vi "WLAN Tx Test Get Default LSL.vi"(8 "error in (no error)":errorcluster, 11 "Template Tx Test in":refnum<class "niDTS WLAN Tx Test.lvclass">) -> (0 "error out":errorcluster, 2 "Default LSL":T1 {"OBW"."Stop Frequency (Hz)" format="%#_4p"; "OBW"."Start Frequency (Hz)" format="%#_4p"; "OBW"."OBW (Hz)" format="%#_4p"}, 3 "Template Tx Test out":refnum<class "niDTS WLAN Tx Test.lvclass">)   [LabVIEW 2015, in "niDTS WLAN.lvlib" / "niDTS WLAN Tx Test.lvclass"]
uses:
  niDTS WLAN Tx Test.lvclass
  Includes/niDTS WLAN Tx Test INC Results.ctl
  Includes/niDTS WLAN Tx Test INC MOD EVM Results.ctl
  Includes/Results/niDTS Tx RES INC EVM.ctl
  Includes/niDTS WLAN Tx Test INC TXP Results.ctl
  Includes/niDTS WLAN Tx Test INC TXP Result SINGLE.ctl
  Includes/niDTS WLAN Tx Test INC OBW Results.ctl
  Instrument/INSTR TX/Results/niDTS WLAN INSTR TX INC SEM Results.ctl
  Instrument/INSTR TX/Results/niDTS WLAN INSTR TX INC SEM FSEGemts Results.ctl
  Includes/Results/niDTS Tx RES INC SEM FSEGemts.ctl
  Instrument/INSTR TX/Results/niDTS WLAN INSTR TX INC SEM MARGin Results.ctl
  Includes/Results/niDTS Tx RES INC SEM Margin.ctl
  Instrument/INSTR TX/Results/niDTS WLAN INSTR TX INC OFDM Impairments Results.ctl
  niDTS WLAN Tx Test.lvclass/niDTS WLAN Tx Test.ctl
  Includes/niDTS WLAN Tx Test INC Default Limits.vi
  niDTS WLAN.lvlib
  Instrument/INSTR TX/niDTS WLAN INSTR TX.lvclass
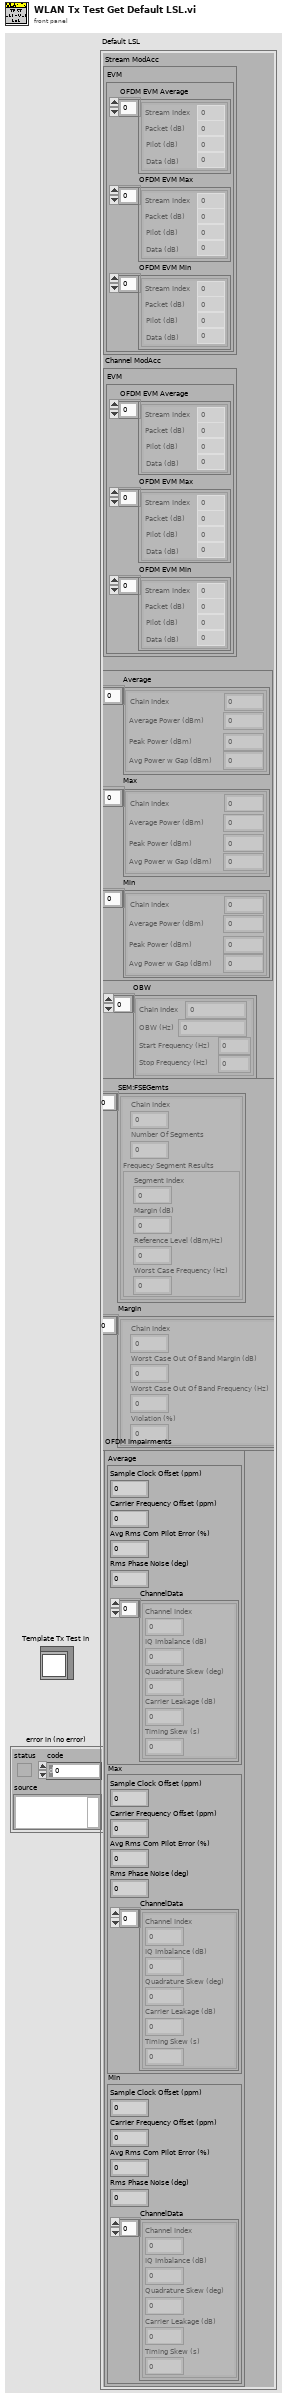
[diagram p1: front panel]
types:
  T1 = typedef "niDTS WLAN.lvlib/niDTS WLAN Tx Test INC Results.ctl" = cluster{"Stream ModAcc":T2, "Channel ModAcc":T2, "TXP":T4, "OBW":T6[], "SEM Results":T7, "OFDM Impairments":T12}
  T2 = typedef "niDTS WLAN.lvlib/niDTS WLAN Tx Test INC MOD EVM Results.ctl" = cluster{"EVM":cluster{"OFDM EVM Average":T3[], "OFDM EVM Max":T3[], "OFDM EVM Min":T3[]}}
  T3 = typedef "niDTS WLAN.lvlib/niDTS Tx RES INC EVM.ctl" = cluster{"Stream Index":i32, "Packet (dB)":dbl, "Pilot (dB)":dbl, "Data (dB)":dbl}
  T4 = typedef "niDTS WLAN.lvlib/niDTS WLAN Tx Test INC TXP Results.ctl" = cluster{"Average":T5[], "Max":T5[], "Min":T5[]}
  T5 = typedef "niDTS WLAN.lvlib/niDTS WLAN Tx Test INC TXP Result SINGLE.ctl" = cluster{"Chain Index":dbl, "Average Power (dBm)":dbl, "Peak Power (dBm)":dbl, "Avg Power w Gap (dBm)":dbl}
  T6 = typedef "niDTS WLAN.lvlib/niDTS WLAN Tx Test INC OBW Results.ctl" = cluster{"Chain Index":dbl, "OBW (Hz)":dbl, "Start Frequency (Hz)":dbl, "Stop Frequency (Hz)":dbl}
  T7 = typedef "niDTS WLAN.lvlib/niDTS WLAN INSTR TX.lvclass/niDTS WLAN INSTR TX INC SEM Results.ctl" = cluster{"SEM:FSEGemts":T8, "Margin":T10}
  T8 = typedef "niDTS WLAN.lvlib/niDTS WLAN INSTR TX.lvclass/niDTS WLAN INSTR TX INC SEM FSEGemts Results.ctl" = T9[]
  T9 = typedef "niDTS WLAN.lvlib/niDTS Tx RES INC SEM FSEGemts.ctl" = cluster{"Chain Index":i32, "Number Of Segments":i32, "Frequecy Segment Results":cluster{"Segment Index":i32, "Margin (dB)":dbl, "Reference Level (dBm/Hz)":dbl, "Worst Case Frequency (Hz)":dbl}}
  T10 = typedef "niDTS WLAN.lvlib/niDTS WLAN INSTR TX.lvclass/niDTS WLAN INSTR TX INC SEM MARGin Results.ctl" = T11[]
  T11 = typedef "niDTS WLAN.lvlib/niDTS Tx RES INC SEM Margin.ctl" = cluster{"Chain Index":i32, "Worst Case Out Of Band Margin (dB)":dbl, "Worst Case Out Of Band Frequency (Hz)":dbl, "Violation (%)":dbl}
  T12 = typedef "niDTS WLAN.lvlib/niDTS WLAN INSTR TX.lvclass/niDTS WLAN INSTR TX INC OFDM Impairments Results.ctl" = cluster{"Average":cluster{"Sample Clock Offset (ppm)":dbl, "Carrier Frequency Offset (ppm)":dbl, "Avg Rms Com Pilot Error (%)":dbl, "Rms Phase Noise (deg)":dbl, "ChannelData":cluster{"Channel Index":i32, "IQ Imbalance (dB)":dbl, "Quadrature Skew (deg)":dbl, "Carrier Leakage (dB)":dbl, "Timing Skew (s)":dbl}[]}, "Max":cluster{"Sample Clock Offset (ppm)":dbl, "Carrier Frequency Offset (ppm)":dbl, "Avg Rms Com Pilot Error (%)":dbl, "Rms Phase Noise (deg)":dbl, "ChannelData":cluster{"Channel Index":i32, "IQ Imbalance (dB)":dbl, "Quadrature Skew (deg)":dbl, "Carrier Leakage (dB)":dbl, "Timing Skew (s)":dbl}[]}, "Min":cluster{"Sample Clock Offset (ppm)":dbl, "Carrier Frequency Offset (ppm)":dbl, "Avg Rms Com Pilot Error (%)":dbl, "Rms Phase Noise (deg)":dbl, "ChannelData":cluster{"Channel Index":i32, "IQ Imbalance (dB)":dbl, "Quadrature Skew (deg)":dbl, "Carrier Leakage (dB)":dbl, "Timing Skew (s)":dbl}[]}}
  T13 = cluster{"OFDM EVM Average":T3[], "OFDM EVM Max":T3[], "OFDM EVM Min":T3[]}
  T14 = typedef "niDTS WLAN.lvlib/niDTS WLAN INC Standard.ctl" = enum16{"802.11 b DSSS", "802.11 a/g OFDM", "802.11 n HT", "802.11 ac VHT"}
  T15 = typedef "niDTS WLAN.lvlib/niDTS WLAN INC CH BW.ctl" = enum16{"20 MHz", "40 MHz", "80 MHz", "160 MHz"}
  T16 = cluster{"SampleClockOffset":dbl, "CarrierFrequencyOffset":dbl, "AvgRmsComPilotErr":dbl, "RmsPhaseNoise":dbl, "ChannelData":cluster{"CarrierFrequencyOffset":i32, "AvgRmsComPilotErr":dbl, "RmsPhaseNoise":dbl, "ChannelData":dbl, "ChannelIndex":dbl}[]}
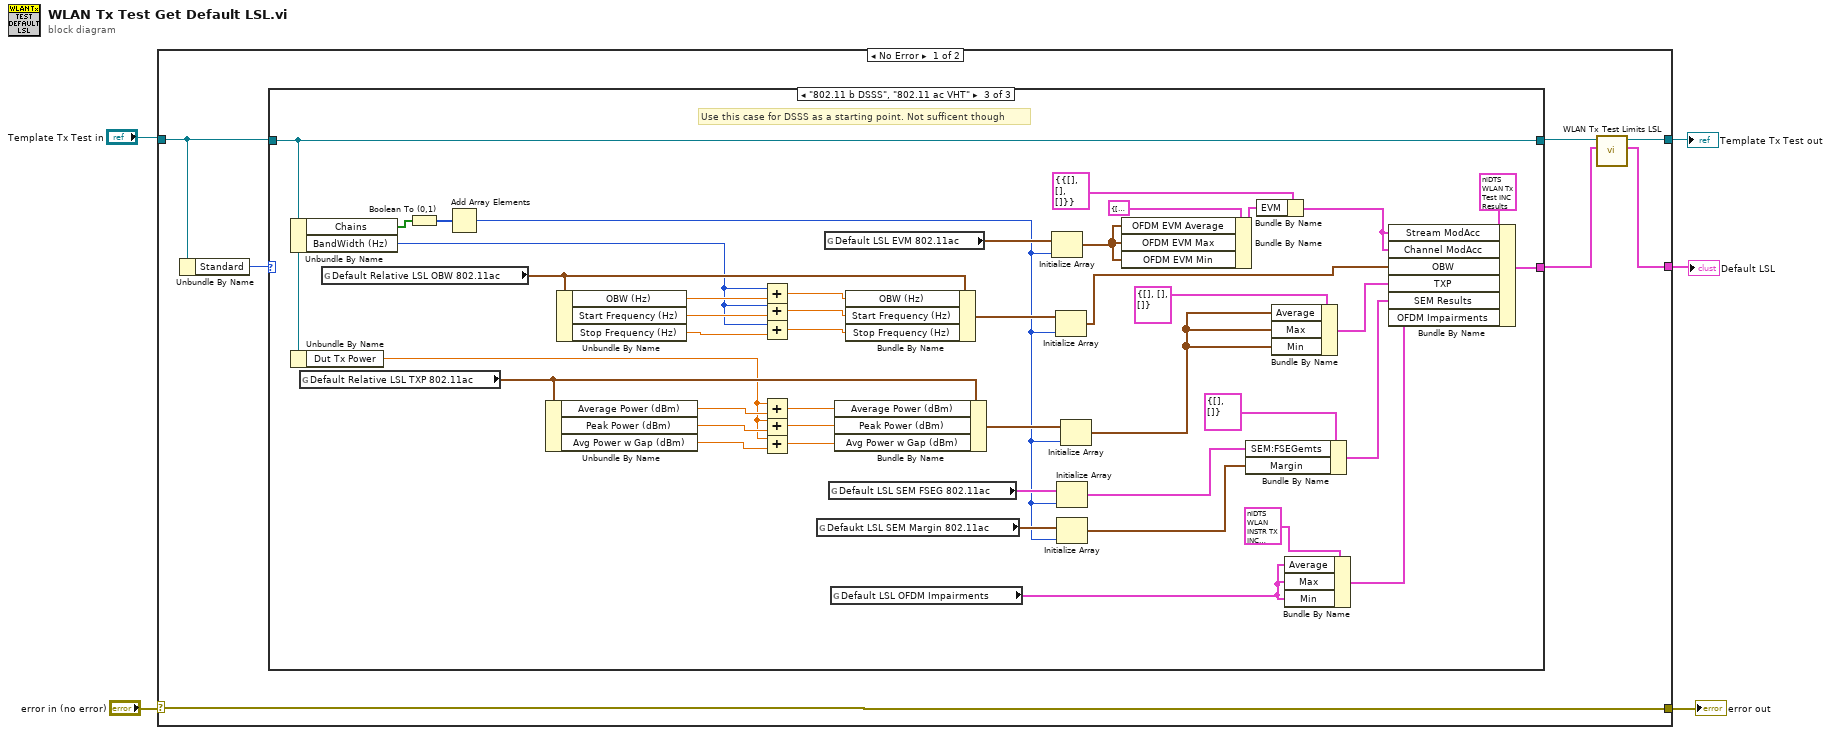
[diagram p0: block diagram]
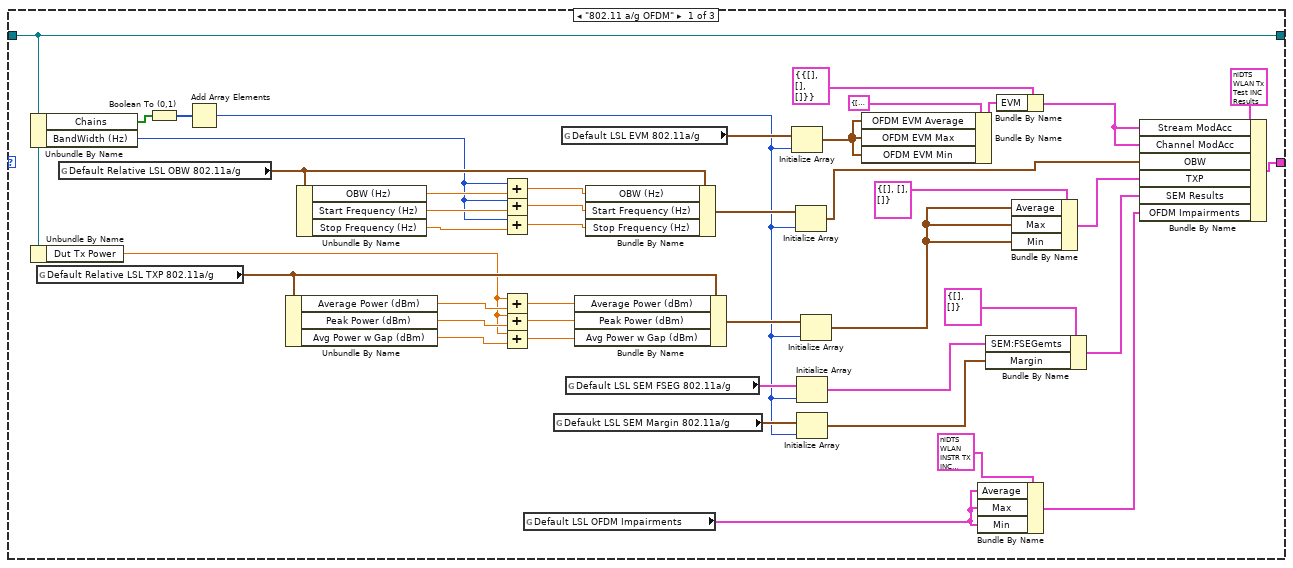
[diagram p2: hidden frame]
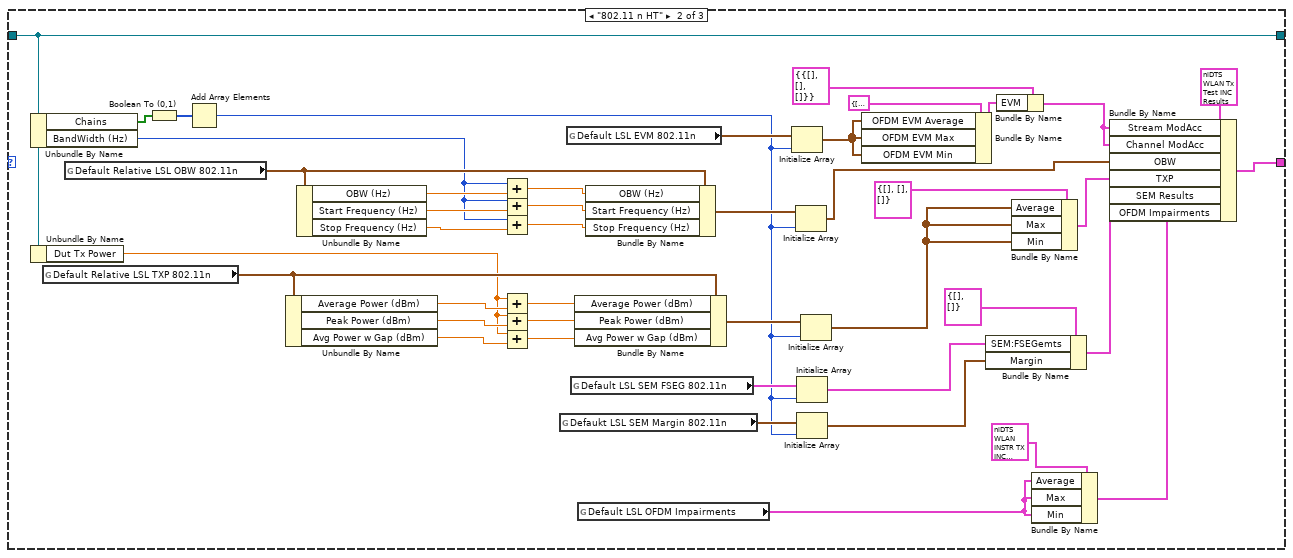
[diagram p3: hidden frame]
diagram:
  n1 = case shown="No Error" "error in (no error)" {
    selector: "error in (no error)" -> [w12 w143]
    tunnel: [w12 w143] -> w1
    tunnel: [w8 w142] -> w3
    tunnel: "Template Tx Test in" -> [w10 w142]
    tunnel: [w6 _] -> w2
    frame No Error {
      n2 = Unbundle By Name(w10) -> ("Standard"=w11:T14)
      n3 = case shown="\"802.11 b DSSS\", \"802.11 ac VHT\"" w11 {
        tunnel: [w54 w97 w140] -> w7
        tunnel: w10 -> [w45 w88 w131]
        tunnel: [w45 w88 w131] -> w9
        frame "802.11 a/g OFDM" {
          n4 = Unbundle By Name(w45) -> ("Chains"=w35:bool[], "BandWidth (Hz)"=w46:T15)
          n5 = Unbundle By Name(w45) -> ("Dut Tx Power"=w37:dbl)
          n6 = global read "niDTS WLAN Tx Test INC Default Limits.vi" "Default Relative LSL TXP 802.11a/g"() -> (w44:T5)
          n7 = global read "niDTS WLAN Tx Test INC Default Limits.vi" "Default Relative LSL OBW 802.11a/g"() -> (w53:T6)
          n8 = Boolean To (0,1)(Boolean=w35) -> (0, 1=w36:i16[])
          n9 = Add Array Elements(numeric array=w36) -> (sum=w18:i16)
          n10 = Unbundle By Name(w44) -> ("Average Power (dBm)"=w43:dbl, "Peak Power (dBm)"=w39:dbl, "Avg Power w Gap (dBm)"=w38:dbl)
          n11 = Unbundle By Name(w53) -> ("OBW (Hz)"=w47:dbl, "Start Frequency (Hz)"=w49:dbl, "Stop Frequency (Hz)"=w48:dbl)
          n12 = Add(x=w46, y=w47) -> (x+y=w52:dbl)
          n13 = Add(x=w46, y=w49) -> (x+y=w51:dbl)
          n14 = Add(x=w46, y=w48) -> (x+y=w50:dbl)
          n15 = Add(x=w37, y=w43) -> (x+y=w42:dbl)
          n16 = Add(x=w37, y=w39) -> (x+y=w41:dbl)
          n17 = Add(x=w37, y=w38) -> (x+y=w40:dbl)
          n18 = global read "niDTS WLAN Tx Test INC Default Limits.vi" "Default LSL OFDM Impairments"() -> (w15:T16)
          n19 = global read "niDTS WLAN Tx Test INC Default Limits.vi" "Defaukt LSL SEM Margin 802.11a/g"() -> (w19:T11)
          n20 = global read "niDTS WLAN Tx Test INC Default Limits.vi" "Default LSL EVM 802.11a/g"() -> (w34:T3)
          n21 = global read "niDTS WLAN Tx Test INC Default Limits.vi" "Default LSL SEM FSEG 802.11a/g"() -> (w21:T9)
          n22 = Bundle By Name(cluster=w44, "Average Power (dBm)"=w42, "Peak Power (dBm)"=w41, "Avg Power w Gap (dBm)"=w40) -> (w25:T5)
          n23 = Bundle By Name(cluster=w53, "OBW (Hz)"=w52, "Start Frequency (Hz)"=w51, "Stop Frequency (Hz)"=w50) -> (w28:T6)
          n24 = Initialize Array(w34, w18) -> (w31:T3[])
          n25 = Initialize Array(w28, w18) -> (w23:T6[])
          n26 = Initialize Array(w21, w18) -> (w20:T9[])
          n27 = Initialize Array(w19, w18) -> (w17:T11[])
          n28 = Initialize Array(w25, w18) -> (w24:T5[])
          n29 = Bundle By Name(cluster=T13 {"OFDM EVM Average"=[], "OFDM EVM Max"=[], "OFDM EVM Min"=[]} ("EVM"), "OFDM EVM Average"=w31, "OFDM EVM Max"=w31, "OFDM EVM Min"=w31) -> (w30:T13)
          n30 = Bundle By Name(cluster=T12 {"Average"={"Sample Clock Offset (ppm)"=0.0, "Carrier Frequency Offset (ppm)"=0.0, "Avg Rms Com Pilot Error (%)"=0.0, "Rms Phase Noise (deg)"=0.0, "ChannelData"=[]}, "Max"={"Sample Clock Offset (ppm)"=0.0, "Carrier Frequency Offset (ppm)"=0.0, "Avg Rms Com Pilot Error (%)"=0.0, "Rms Phase Noise (deg)"=0.0, "ChannelData"=[]}, "Min"={"Sample Clock Offset (ppm)"=0.0, "Carrier Frequency Offset (ppm)"=0.0, "Avg Rms Com Pilot Error (%)"=0.0, "Rms Phase Noise (deg)"=0.0, "ChannelData"=[]}} ("OFDM Impairments"), "Average"=w15, "Max"=w15, "Min"=w15) -> (w13:T12)
          n31 = Bundle By Name(cluster=T7 {"SEM:FSEGemts"=[], "Margin"=[]} ("SEM Results"), "SEM:FSEGemts"=w20, "Margin"=w17) -> (w16:T7)
          n32 = Bundle By Name(cluster=T2 {"EVM"={"OFDM EVM Average"=[], "OFDM EVM Max"=[], "OFDM EVM Min"=[]}} ("Stream ModAcc"), "EVM"=w30) -> (w29:T2)
          n33 = Bundle By Name(cluster=T4 {"Average"=[], "Max"=[], "Min"=[]} ("TXP Results"), "Average"=w24, "Max"=w24, "Min"=w24) -> (w26:T4)
          n34 = Bundle By Name(cluster=T1 {"Stream ModAcc"={"EVM"={"OFDM EVM Average"=[], "OFDM EVM Max"=[], "OFDM EVM Min"=[]}}, "Channel ModAcc"={"EVM"={"OFDM EVM Average"=[], "OFDM EVM Max"=[], "OFDM EVM Min"=[]}}, "TXP"={"Average"=[], "Max"=[], "Min"=[]}, "OBW"=[], "SEM Results"={"SEM:FSEGemts"=[], "Margin"=[]}, "OFDM Impairments"={"Average"={"Sample Clock Offset (ppm)"=0.0, "Carrier Frequency Offset (ppm)"=0.0, "Avg Rms Com Pilot Error (%)"=0.0, "Rms Phase Noise (deg)"=0.0, "ChannelData"=[]}, "Max"={"Sample Clock Offset (ppm)"=0.0, "Carrier Frequency Offset (ppm)"=0.0, "Avg Rms Com Pilot Error (%)"=0.0, "Rms Phase Noise (deg)"=0.0, "ChannelData"=[]}, "Min"={"Sample Clock Offset (ppm)"=0.0, "Carrier Frequency Offset (ppm)"=0.0, "Avg Rms Com Pilot Error (%)"=0.0, "Rms Phase Noise (deg)"=0.0, "ChannelData"=[]}}} ("Default USL"), "Stream ModAcc"=w29, "Channel ModAcc"=w29, "OBW"=w23, "TXP"=w26, "SEM Results"=w16, "OFDM Impairments"=w13) -> (w54:T1)
        }
        frame "802.11 n HT" {
          n35 = Unbundle By Name(w88) -> ("Chains"=w78:bool[], "BandWidth (Hz)"=w89:T15)
          n36 = Unbundle By Name(w88) -> ("Dut Tx Power"=w80:dbl)
          n37 = global read "niDTS WLAN Tx Test INC Default Limits.vi" "Default Relative LSL TXP 802.11n"() -> (w87:T5)
          n38 = global read "niDTS WLAN Tx Test INC Default Limits.vi" "Default Relative LSL OBW 802.11n"() -> (w96:T6)
          n39 = Boolean To (0,1)(Boolean=w78) -> (0, 1=w79:i16[])
          n40 = Add Array Elements(numeric array=w79) -> (sum=w61:i16)
          n41 = Unbundle By Name(w87) -> ("Average Power (dBm)"=w86:dbl, "Peak Power (dBm)"=w82:dbl, "Avg Power w Gap (dBm)"=w81:dbl)
          n42 = Unbundle By Name(w96) -> ("OBW (Hz)"=w90:dbl, "Start Frequency (Hz)"=w92:dbl, "Stop Frequency (Hz)"=w91:dbl)
          n43 = Add(x=w89, y=w90) -> (x+y=w95:dbl)
          n44 = Add(x=w89, y=w92) -> (x+y=w94:dbl)
          n45 = Add(x=w89, y=w91) -> (x+y=w93:dbl)
          n46 = Add(x=w80, y=w86) -> (x+y=w85:dbl)
          n47 = Add(x=w80, y=w82) -> (x+y=w84:dbl)
          n48 = Add(x=w80, y=w81) -> (x+y=w83:dbl)
          n49 = global read "niDTS WLAN Tx Test INC Default Limits.vi" "Defaukt LSL SEM Margin 802.11n"() -> (w62:T11)
          n50 = global read "niDTS WLAN Tx Test INC Default Limits.vi" "Default LSL EVM 802.11n"() -> (w77:T3)
          n51 = global read "niDTS WLAN Tx Test INC Default Limits.vi" "Default LSL SEM FSEG 802.11n"() -> (w64:T9)
          n52 = Bundle By Name(cluster=w87, "Average Power (dBm)"=w85, "Peak Power (dBm)"=w84, "Avg Power w Gap (dBm)"=w83) -> (w68:T5)
          n53 = global read "niDTS WLAN Tx Test INC Default Limits.vi" "Default LSL OFDM Impairments"() -> (w57:T16)
          n54 = Bundle By Name(cluster=w96, "OBW (Hz)"=w95, "Start Frequency (Hz)"=w94, "Stop Frequency (Hz)"=w93) -> (w71:T6)
          n55 = Initialize Array(w77, w61) -> (w74:T3[])
          n56 = Initialize Array(w71, w61) -> (w66:T6[])
          n57 = Initialize Array(w64, w61) -> (w63:T9[])
          n58 = Initialize Array(w62, w61) -> (w60:T11[])
          n59 = Initialize Array(w68, w61) -> (w67:T5[])
          n60 = Bundle By Name(cluster=T13 {"OFDM EVM Average"=[], "OFDM EVM Max"=[], "OFDM EVM Min"=[]} ("EVM"), "OFDM EVM Average"=w74, "OFDM EVM Max"=w74, "OFDM EVM Min"=w74) -> (w73:T13)
          n61 = Bundle By Name(cluster=T7 {"SEM:FSEGemts"=[], "Margin"=[]} ("SEM Results"), "SEM:FSEGemts"=w63, "Margin"=w60) -> (w59:T7)
          n62 = Bundle By Name(cluster=T2 {"EVM"={"OFDM EVM Average"=[], "OFDM EVM Max"=[], "OFDM EVM Min"=[]}} ("Stream ModAcc"), "EVM"=w73) -> (w72:T2)
          n63 = Bundle By Name(cluster=T4 {"Average"=[], "Max"=[], "Min"=[]} ("TXP Results"), "Average"=w67, "Max"=w67, "Min"=w67) -> (w69:T4)
          n64 = Bundle By Name(cluster=T12 {"Average"={"Sample Clock Offset (ppm)"=0.0, "Carrier Frequency Offset (ppm)"=0.0, "Avg Rms Com Pilot Error (%)"=0.0, "Rms Phase Noise (deg)"=0.0, "ChannelData"=[]}, "Max"={"Sample Clock Offset (ppm)"=0.0, "Carrier Frequency Offset (ppm)"=0.0, "Avg Rms Com Pilot Error (%)"=0.0, "Rms Phase Noise (deg)"=0.0, "ChannelData"=[]}, "Min"={"Sample Clock Offset (ppm)"=0.0, "Carrier Frequency Offset (ppm)"=0.0, "Avg Rms Com Pilot Error (%)"=0.0, "Rms Phase Noise (deg)"=0.0, "ChannelData"=[]}} ("OFDM Impairments"), "Average"=w57, "Max"=w57, "Min"=w57) -> (w56:T12)
          n65 = Bundle By Name(cluster=T1 {"Stream ModAcc"={"EVM"={"OFDM EVM Average"=[], "OFDM EVM Max"=[], "OFDM EVM Min"=[]}}, "Channel ModAcc"={"EVM"={"OFDM EVM Average"=[], "OFDM EVM Max"=[], "OFDM EVM Min"=[]}}, "TXP"={"Average"=[], "Max"=[], "Min"=[]}, "OBW"=[], "SEM Results"={"SEM:FSEGemts"=[], "Margin"=[]}, "OFDM Impairments"={"Average"={"Sample Clock Offset (ppm)"=0.0, "Carrier Frequency Offset (ppm)"=0.0, "Avg Rms Com Pilot Error (%)"=0.0, "Rms Phase Noise (deg)"=0.0, "ChannelData"=[]}, "Max"={"Sample Clock Offset (ppm)"=0.0, "Carrier Frequency Offset (ppm)"=0.0, "Avg Rms Com Pilot Error (%)"=0.0, "Rms Phase Noise (deg)"=0.0, "ChannelData"=[]}, "Min"={"Sample Clock Offset (ppm)"=0.0, "Carrier Frequency Offset (ppm)"=0.0, "Avg Rms Com Pilot Error (%)"=0.0, "Rms Phase Noise (deg)"=0.0, "ChannelData"=[]}}} ("Default USL"), "Stream ModAcc"=w72, "Channel ModAcc"=w72, "OBW"=w66, "TXP"=w69, "SEM Results"=w59, "OFDM Impairments"=w56) -> (w97:T1)
        }
        frame "802.11 b DSSS", "802.11 ac VHT" {
          # "Use this case for DSSS as a starting point. Not sufficent though"
          n66 = Unbundle By Name(w131) -> ("Chains"=w121:bool[], "BandWidth (Hz)"=w132:T15)
          n67 = Unbundle By Name(w131) -> ("Dut Tx Power"=w123:dbl)
          n68 = global read "niDTS WLAN Tx Test INC Default Limits.vi" "Default Relative LSL TXP 802.11ac"() -> (w130:T5)
          n69 = global read "niDTS WLAN Tx Test INC Default Limits.vi" "Default Relative LSL OBW 802.11ac"() -> (w139:T6)
          n70 = Boolean To (0,1)(Boolean=w121) -> (0, 1=w122:i16[])
          n71 = Add Array Elements(numeric array=w122) -> (sum=w104:i16)
          n72 = Unbundle By Name(w130) -> ("Average Power (dBm)"=w129:dbl, "Peak Power (dBm)"=w125:dbl, "Avg Power w Gap (dBm)"=w124:dbl)
          n73 = Unbundle By Name(w139) -> ("OBW (Hz)"=w133:dbl, "Start Frequency (Hz)"=w135:dbl, "Stop Frequency (Hz)"=w134:dbl)
          n74 = Add(x=w132, y=w133) -> (x+y=w138:dbl)
          n75 = Add(x=w132, y=w135) -> (x+y=w137:dbl)
          n76 = Add(x=w132, y=w134) -> (x+y=w136:dbl)
          n77 = Add(x=w123, y=w129) -> (x+y=w128:dbl)
          n78 = Add(x=w123, y=w125) -> (x+y=w127:dbl)
          n79 = Add(x=w123, y=w124) -> (x+y=w126:dbl)
          n80 = global read "niDTS WLAN Tx Test INC Default Limits.vi" "Defaukt LSL SEM Margin 802.11ac"() -> (w105:T11)
          n81 = global read "niDTS WLAN Tx Test INC Default Limits.vi" "Default LSL EVM 802.11ac"() -> (w120:T3)
          n82 = global read "niDTS WLAN Tx Test INC Default Limits.vi" "Default LSL SEM FSEG 802.11ac"() -> (w107:T9)
          n83 = global read "niDTS WLAN Tx Test INC Default Limits.vi" "Default LSL OFDM Impairments"() -> (w99:T16)
          n84 = Bundle By Name(cluster=w130, "Average Power (dBm)"=w128, "Peak Power (dBm)"=w127, "Avg Power w Gap (dBm)"=w126) -> (w111:T5)
          n85 = Bundle By Name(cluster=w139, "OBW (Hz)"=w138, "Start Frequency (Hz)"=w137, "Stop Frequency (Hz)"=w136) -> (w114:T6)
          n86 = Initialize Array(w120, w104) -> (w117:T3[])
          n87 = Initialize Array(w114, w104) -> (w109:T6[])
          n88 = Initialize Array(w107, w104) -> (w106:T9[])
          n89 = Initialize Array(w105, w104) -> (w103:T11[])
          n90 = Initialize Array(w111, w104) -> (w110:T5[])
          n91 = Bundle By Name(cluster=T13 {"OFDM EVM Average"=[], "OFDM EVM Max"=[], "OFDM EVM Min"=[]} ("EVM"), "OFDM EVM Average"=w117, "OFDM EVM Max"=w117, "OFDM EVM Min"=w117) -> (w116:T13)
          n92 = Bundle By Name(cluster=T7 {"SEM:FSEGemts"=[], "Margin"=[]} ("SEM Results"), "SEM:FSEGemts"=w106, "Margin"=w103) -> (w102:T7)
          n93 = Bundle By Name(cluster=T2 {"EVM"={"OFDM EVM Average"=[], "OFDM EVM Max"=[], "OFDM EVM Min"=[]}} ("Stream ModAcc"), "EVM"=w116) -> (w115:T2)
          n94 = Bundle By Name(cluster=T4 {"Average"=[], "Max"=[], "Min"=[]} ("TXP Results"), "Average"=w110, "Max"=w110, "Min"=w110) -> (w112:T4)
          n95 = Bundle By Name(cluster=T12 {"Average"={"Sample Clock Offset (ppm)"=0.0, "Carrier Frequency Offset (ppm)"=0.0, "Avg Rms Com Pilot Error (%)"=0.0, "Rms Phase Noise (deg)"=0.0, "ChannelData"=[]}, "Max"={"Sample Clock Offset (ppm)"=0.0, "Carrier Frequency Offset (ppm)"=0.0, "Avg Rms Com Pilot Error (%)"=0.0, "Rms Phase Noise (deg)"=0.0, "ChannelData"=[]}, "Min"={"Sample Clock Offset (ppm)"=0.0, "Carrier Frequency Offset (ppm)"=0.0, "Avg Rms Com Pilot Error (%)"=0.0, "Rms Phase Noise (deg)"=0.0, "ChannelData"=[]}} ("OFDM Impairments"), "Average"=w99, "Max"=w99, "Min"=w99) -> (w101:T12)
          n96 = Bundle By Name(cluster=T1 {"Stream ModAcc"={"EVM"={"OFDM EVM Average"=[], "OFDM EVM Max"=[], "OFDM EVM Min"=[]}}, "Channel ModAcc"={"EVM"={"OFDM EVM Average"=[], "OFDM EVM Max"=[], "OFDM EVM Min"=[]}}, "TXP"={"Average"=[], "Max"=[], "Min"=[]}, "OBW"=[], "SEM Results"={"SEM:FSEGemts"=[], "Margin"=[]}, "OFDM Impairments"={"Average"={"Sample Clock Offset (ppm)"=0.0, "Carrier Frequency Offset (ppm)"=0.0, "Avg Rms Com Pilot Error (%)"=0.0, "Rms Phase Noise (deg)"=0.0, "ChannelData"=[]}, "Max"={"Sample Clock Offset (ppm)"=0.0, "Carrier Frequency Offset (ppm)"=0.0, "Avg Rms Com Pilot Error (%)"=0.0, "Rms Phase Noise (deg)"=0.0, "ChannelData"=[]}, "Min"={"Sample Clock Offset (ppm)"=0.0, "Carrier Frequency Offset (ppm)"=0.0, "Avg Rms Com Pilot Error (%)"=0.0, "Rms Phase Noise (deg)"=0.0, "ChannelData"=[]}}} ("Default USL"), "Stream ModAcc"=w115, "Channel ModAcc"=w115, "OBW"=w109, "TXP"=w112, "SEM Results"=w102, "OFDM Impairments"=w101) -> (w140:T1)
        }
      }
      n97 = call "WLAN Tx Test Limits LSL.vi"("Limits"=w7, "WLAN Tx Test in"=w9) -> ("Limits Out"=w6:T1, "WLAN Tx Test out"=w8:refnum<class "niDTS WLAN Tx Test.lvclass">)  [unwired: 7 in, 1 out]
    }
    frame Error {
    }
  }
  "error out" <- w1
  "Template Tx Test out" <- w3
  "Default LSL" <- w2
